vi "Untitled 2.vi"() -> ()   [LabVIEW 2012]
panel:
  in  "stop":bool
  in  "WM_Switch":bool
  in  "Cancel":bool
  in  "Off_Line":bool
  in  "On_Line":bool
  out "LockStat_Out":T1
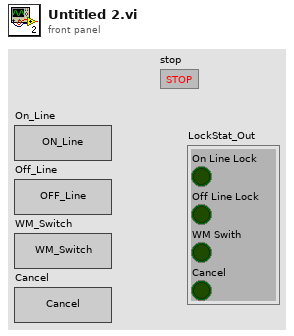
[diagram p1: front panel]
types:
  T1 = cluster{"On Line Lock":bool, "Off Line Lock":bool, "WM Swith":bool, "Cancel":bool}
  T2 = enum16{"LS_Init", "LS_Read", "On_Line", "Off_line", "WM_Switch", "Cancel"}
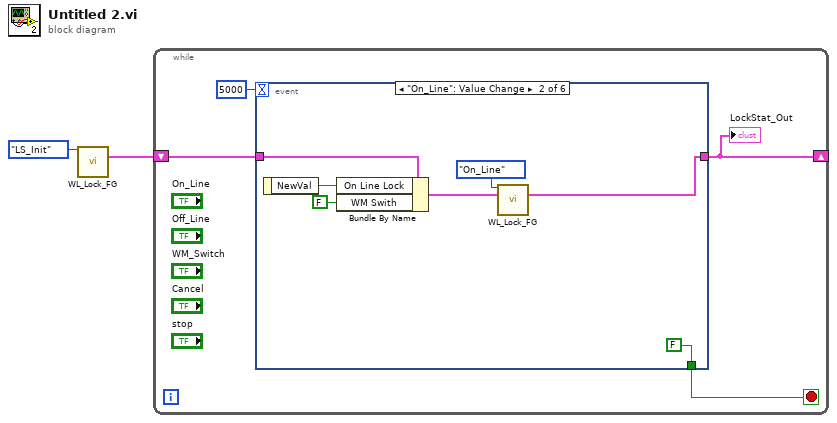
[diagram p0: block diagram]
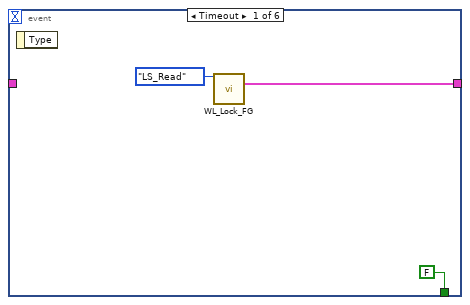
[diagram p2: hidden frame]
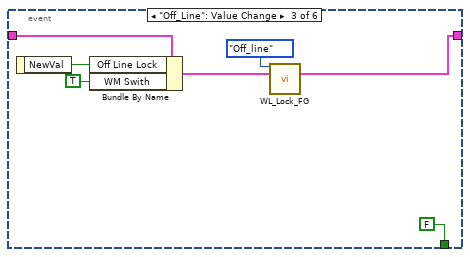
[diagram p3: hidden frame]
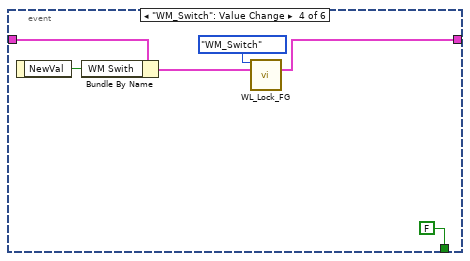
[diagram p4: hidden frame]
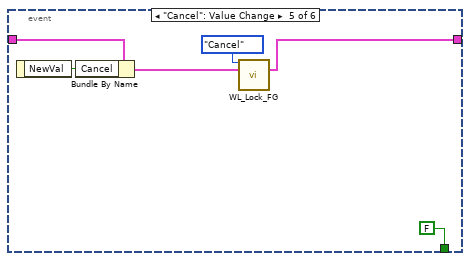
[diagram p5: hidden frame]
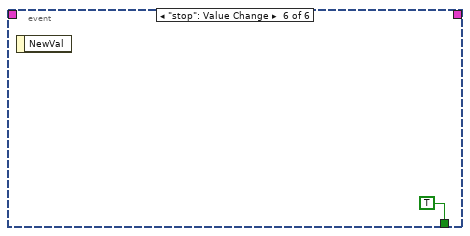
[diagram p6: hidden frame]
diagram:
  n1 = call "WL_Lock_FG.vi"("Command"=T2."LS_Init") -> ("LockStat_Out"=w1:T1)  [unwired: 13 in, 1 out]
  n2 = while {
    shift-right: [w4] -> _
    shift-left: w1 -> [w5]
    stop <- w3 stop-if-true
    n3 = event shown="[1] \"On_Line\": Value Change" {
      selector: _ -> [_ _ _ _ _ _]
      dyn-events: _ -> [_ _ _ _ _ _]
      timeout: 5000 -> [_ _ _ _ _ _]
      tunnel: w5 -> [_ w16 w23 w28 w34 _]
      tunnel: [w8 w13 w20 w25 w31 _] -> w4
      tunnel: [FALSE FALSE FALSE FALSE FALSE TRUE] -> w3
      event Timeout {
        n4 = event-data() -> ()  [unwired: 1 in, 1 out]
        n5 = call "WL_Lock_FG.vi"("Command"=T2."LS_Read") -> ("LockStat_Out"=w8:T1)  [unwired: 13 in, 1 out]
      }
      event "On_Line": Value Change {
        n6 = event-data() -> ("NewVal"=w15:bool)  [unwired: 1 in]
        n7 = Bundle By Name(cluster=w16, "On Line Lock"=w15, "WM Swith"=FALSE) -> (w14:T1)
        n8 = call "WL_Lock_FG.vi"("Command"=T2."On_Line", "LockStat_In"=w14) -> ("LockStat_Out"=w13:T1)  [unwired: 12 in, 1 out]
      }
      event "Off_Line": Value Change {
        n9 = event-data() -> ("NewVal"=w22:bool)  [unwired: 1 in]
        n10 = Bundle By Name(cluster=w23, "Off Line Lock"=w22, "WM Swith"=TRUE) -> (w21:T1)
        n11 = call "WL_Lock_FG.vi"("Command"=T2."Off_line", "LockStat_In"=w21) -> ("LockStat_Out"=w20:T1)  [unwired: 12 in, 1 out]
      }
      event "WM_Switch": Value Change {
        n12 = event-data() -> ("NewVal"=w29:bool)  [unwired: 1 in]
        n13 = Bundle By Name(cluster=w28, "WM Swith"=w29) -> (w27:T1)
        n14 = call "WL_Lock_FG.vi"("Command"=T2."WM_Switch", "LockStat_In"=w27) -> ("LockStat_Out"=w25:T1)  [unwired: 12 in, 1 out]
      }
      event "Cancel": Value Change {
        n15 = event-data() -> ("NewVal"=w35:bool)  [unwired: 1 in]
        n16 = Bundle By Name(cluster=w34, "Cancel"=w35) -> (w33:T1)
        n17 = call "WL_Lock_FG.vi"("Command"=T2."Cancel", "LockStat_In"=w33) -> ("LockStat_Out"=w31:T1)  [unwired: 12 in, 1 out]
      }
      event "stop": Value Change {
        n18 = event-data() -> ()  [unwired: 1 in, 1 out]
      }
    }
    "LockStat_Out" <- w4
  }
